vi "Start Data Save.vi"(7 "Generate Index":bool=TRUE, 8 "error in (no error)":errorcluster, 10 "Save data details":T3, 11 "Save data settings":T1={"Save data"=TRUE, "Data Root Path"=path "", "File Prefix"="", "File Format"=enum."ASCII", "Save column names"=TRUE, "File Comments"="<Description of the current file>", "User/Prj"="<User Name/Project Description>"}) -> (0 "error out":errorcluster, 2 "Save data details out":T3, 3 "Save data settings out":T1={"Save data"=TRUE, "Data Root Path"=path "", "File Prefix"="", "File Format"=enum."ASCII", "Save column names"=TRUE, "File Comments"="<Description of the current file>", "User/Prj"="<User Name/Project Description>"})   [LabVIEW 2015]
uses:
  Controls/Save data settings.ctl
  Controls/File formats.ctl
  Controls/Save data details.ctl
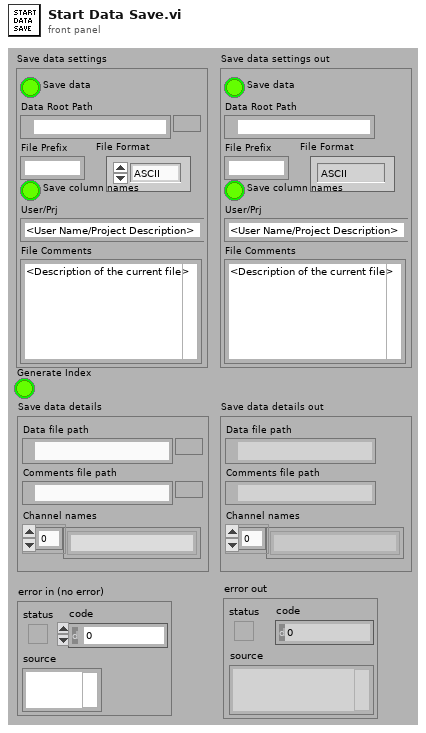
[diagram p1: front panel]
types:
  T1 = typedef "Save data settings.ctl" = cluster{"Save data":bool, "Data Root Path":path, "File Prefix":string, "File Format":T2, "Save column names":bool, "File Comments":string, "User/Prj":string}
  T2 = typedef "File formats.ctl" = enum16{"TDMS", "ASCII", "BINARY"}
  T3 = typedef "Save data details.ctl" = cluster{"Data file path":path, "Comments file path":path, "Channel names":string[]}
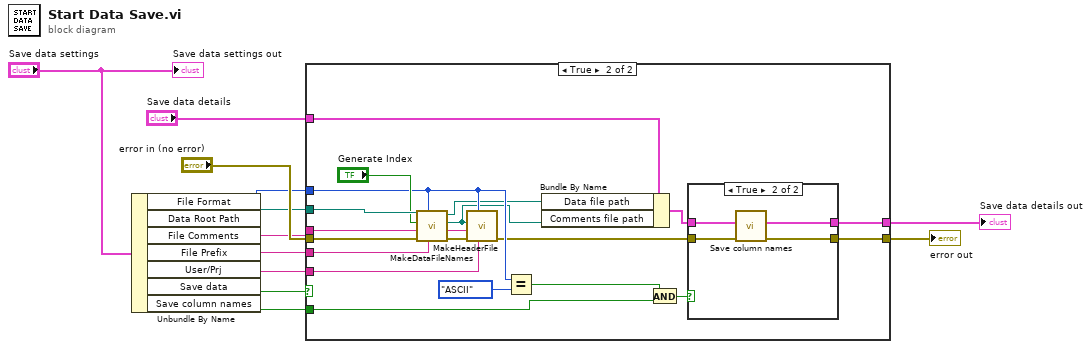
[diagram p0: block diagram]
diagram:
  n1 = Unbundle By Name("Save data settings") -> ("File Format"=w7:T2, "Data Root Path"=w10:path, "File Comments"=w11:string, "File Prefix"=w8:string, "User/Prj"=w9:string, "Save data"=w6:bool, "Save column names"=w3:bool)
  n2 = case shown="True" w6 {
    tunnel: "error in (no error)" -> [w14 w29]
    tunnel: [w14 w20] -> w5
    tunnel: w10 -> [_ w31]
    tunnel: w8 -> [_ w30]
    tunnel: w11 -> [_ w33]
    tunnel: w9 -> [_ w32]
    tunnel: w7 -> [_ w26]
    tunnel: w3 -> [_ w23]
    tunnel: "Save data details" -> [w13 w16]
    tunnel: [w13 w15] -> w1
    frame False {
    }
    frame True {
      n3 = call "MakeDataFileNames.vi"("File Prefix"=w30, "File format"=w26, "Error In"=w29, "Generate Index"="Generate Index", "Root Data Folder"=w31) -> ("Error Out"=w28:errorcluster, "Settings File Path"=w18:path, "Data File  Path"=w19:path)  [unwired: 3 in, 1 out]
      n4 = call "MakeHeaderFile.vi"("Parameters"=w32, "File Format"=w26, "error in (no error)"=w28, "File Description"=w33, "File Name"=w18) -> ("error out"=w21:errorcluster)  [unwired: 4 in, 2 out]
      n5 = Equal?(x=w26, y=File_formats."ASCII") -> (x = y?=w24:bool)
      n6 = Bundle By Name(cluster=w16, "Data file path"=w19, "Comments file path"=w18) -> (w17:T3)
      n7 = And(x=w24, y=w23) -> (x .and. y?=w22:bool)
      n8 = case shown="True" w22 {
        tunnel: w21 -> [w34 w39]
        tunnel: [w34 w38] -> w20
        tunnel: w17 -> [w35 w37]
        tunnel: [w35 w36] -> w15
        frame False {
        }
        frame True {
          n9 = call "Save column names.vi"("error in (no error)"=w39, "Save data details"=w37) -> ("error out"=w38:errorcluster, "Save data details out"=w36:T3)  [unwired: 8 in]
        }
      }
    }
  }
  "error out" <- w5
  "Save data details out" <- w1
  "Save data settings out" <- "Save data settings"
